vi "Single GPIO.vi"() -> ()   [LabVIEW 2020, in "CTI-Visa-Scratchpad.lvlib"]
uses:
  CTI-Visa-Scratchpad.lvlib
  CTI-Visa/Digital Direction.ctl
  CTI-Visa/CTI-Visa.lvlib
panel:
  in  "Channel":i32
  out "Readback":bool
  in  "Control":bool
  in  "Port":refnum<visa-resource-name>="COM3"
  in  "stop":bool
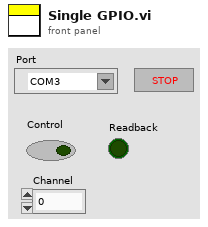
[diagram p1: front panel]
types:
  T1 = typedef "CTI-Visa.lvlib/Digital Direction.ctl" = enum16{"In", "Out"}
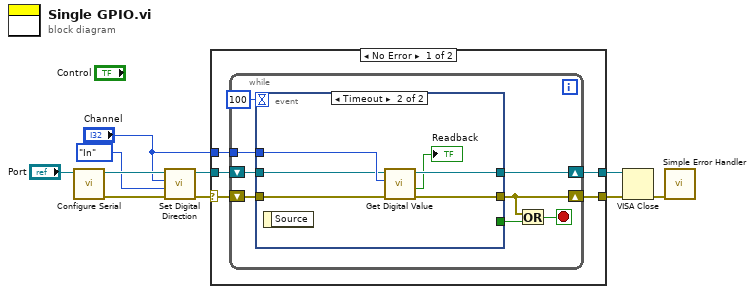
[diagram p0: block diagram]
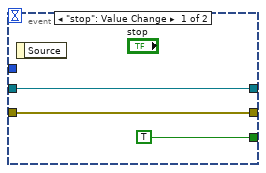
[diagram p2: hidden frame]
diagram:
  n1 = call "Configure Serial.vi"("VISA resource name in"="Port") -> ("error out"=w8:errorcluster, "VISA resource name"=w9:refnum<visa-resource-name>)  [unwired: 9 in]
  n2 = call "Set Digital Direction.vi"("error in (no error)"=w8, "Direction"=Digital_Direction."In", "Channel"="Channel", "VISA resource name in"=w9) -> ("error out"=w6:errorcluster, "VISA resource name"=w7:refnum<visa-resource-name>)  [unwired: 6 in]
  n3 = case shown="No Error" w6 {
    selector: w6 -> [w14 w33]
    tunnel: w7 -> [w15 w34]
    tunnel: [w13 w34] -> w5
    tunnel: [w12 w33] -> w4
    tunnel: "Channel" -> [w11 _]
    frame No Error {
      n4 = while {
        shift-right: [w21] -> w13
        shift-left: w15 -> [w23]
        shift-right: [w20] -> w12
        shift-left: w14 -> [w22]
        tunnel: w11 -> [w17]
        stop <- w19 stop-if-true
        n5 = event shown="[1] Timeout" {
          selector: _ -> [_ _]
          dyn-events: _ -> [_ _]
          timeout: 100 -> [_ _]
          tunnel: w23 -> [w26 w28]
          tunnel: w22 -> [w25 w27]
          tunnel: [w26 w32] -> w21
          tunnel: [w25 w31] -> w20
          tunnel: [TRUE _] -> w18
          tunnel: w17 -> [_ w29]
          event "stop": Value Change {
            n6 = event-data() -> ()  [unwired: 1 in, 1 out]
          }
          event Timeout {
            n7 = event-data() -> ()  [unwired: 1 in, 1 out]
            n8 = call "Get Digital Value.vi"("error in (no error)"=w27, "Channel"=w29, "VISA resource name in"=w28) -> ("error out"=w31:errorcluster, "Value"=→"Readback":bool, "VISA resource name"=w32:refnum<visa-resource-name>)  [unwired: 6 in]
          }
        }
        n9 = Or(x=w20, y=w18) -> (x .or. y?=w19:bool)
      }
    }
    frame Error {
    }
  }
  n10 = VISA Close(VISA resource name=w5, error in (no error)=w4) -> (error out=w3:errorcluster)
  n11 = call <vilib>:"Simple Error Handler.vi"("error in (no error)"=w3) -> ()  [unwired: 4 in, 5 out]
